vi "Config Type.vi"(11 "OutOfRange Condition in":refnum<class "OutOfRange Condition.lvclass">) -> (2 "Condition Config":refnum<class "Condition Config.lvclass">)   [LabVIEW 2020, in "VolatusSeq.lvlib" / "OutOfRange Condition.lvclass"]
uses:
  OutOfRange Condition.lvclass
  OutOfRange Condition.lvclass/OutOfRange Condition.ctl
  VolatusSeqConfig/OutOfRange Condition Config/OutOfRange Condition Config.lvclass
  C:/dev/lv20CE/relink/lv-volatus/VolatusSeqConfig/Condition Config/Condition Config.lvclass
  C:/dev/lv20CE/relink/lv-volatus/VolatusSeqConfig/OutOfRange Condition Config/OutOfRange Condition Config.lvclass
  VolatusSeqConfig/Condition Config/Condition Config.lvclass
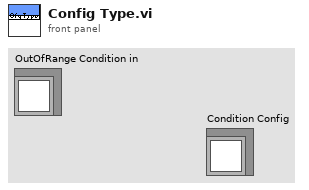
[diagram p1: front panel]
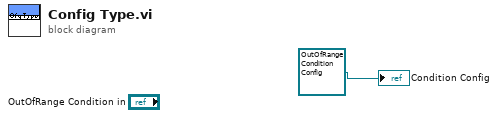
[diagram p0: block diagram]
diagram:
  "Condition Config" <- refnum<class "OutOfRange Condition Config.lvclass"> refnum ("VolatusSeqConfig.lvlib:OutOfRange Condition Config.lvclass")
